vi "Set Pump Enable.vi"(8 "Error in":errorcluster caption="错误输入", 9 "Enable":u16(ring) caption="使能" items=["禁止", "使能"], 10 "Channel":dbl=1.0 caption="设备通道", 11 "Modbus instance in":refnum<class "Modbus API.lvclass"> caption="Modbus实例输入") -> (0 "Error out":errorcluster caption="错误输出", 3 "Modbus instance out":refnum<class "Modbus API.lvclass"> caption="Modbus实例输出")   [LabVIEW 2023, in "Longer Pump dLSP501 Series.lvlib"]
uses:
  <instrlib>/Longer Pump dLSP501 Modbus RTU Series/Longer Pump dLSP501 Series.lvlib
  <vilib>/NI/Modbus Library/API/Modbus API.lvclass
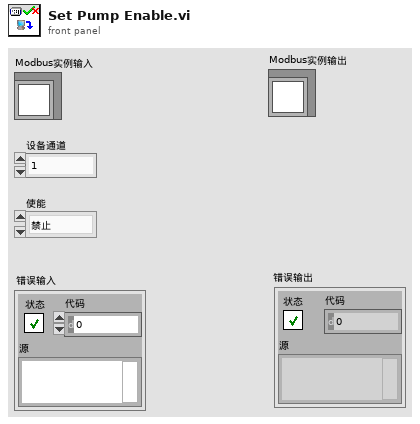
[diagram p1: front panel]
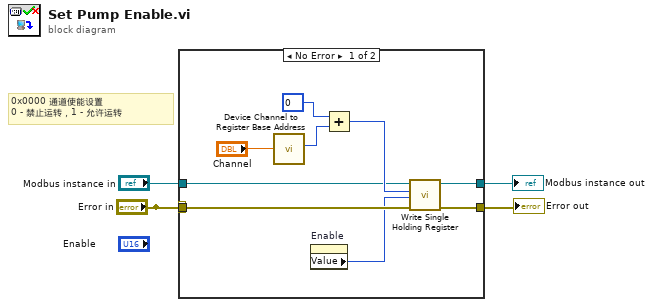
[diagram p0: block diagram]
diagram:
  # "0x0000\t通道使能设置\n0 - 禁止运转，1 - 允许运转"
  n1 = case shown="No Error" "Error in" {
    selector: "Error in" -> [_ w14]
    tunnel: "Error in" -> [w13 _]
    tunnel: "Modbus instance in" -> [w5 w15]
    tunnel: [w12 w14] -> w2
    tunnel: [w11 w15] -> w3
    frame No Error {
      n2 = call <instrlib>:"Device Channel to Register Base Address.vi"("Channel"="Channel") -> ("Register Base Address"=w8:u16)  [unwired: 10 in]
      n3 = property on="Enable" class="Ring (strict)"() -> ("Value"=w10:u16)  [unwired: 2 in, 2 out]
      n4 = Add(x=u16 0 ("address"), y=w8) -> (x+y=w6:u16)
      n5 = call-dynamic "Write Single Holding Register.vi"("error in"=w13, "register to write"=w10, "address"=w6, "Modbus instance in"=w5) -> ("error out"=w12:errorcluster, "Modbus instance out"=w11:refnum<class "Modbus API.lvclass">)  [unwired: 6 in]
    }
    frame Error {
    }
  }
  "Modbus instance out" <- w3
  "Error out" <- w2
